vi "Get Board Size.vi"(10 "Board":u32[][](array[colorbox])) -> (1 "Y":i32, 2 "X":i32)   [LabVIEW 2021, in "Board_Game.lvclass"]
uses:
  Board_Game.lvclass
  Board_Game.lvclass/Board_Game.ctl
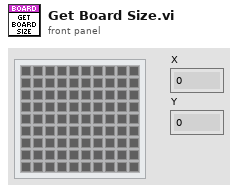
[diagram p1: front panel]
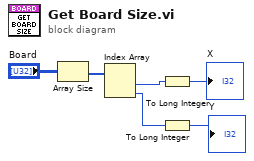
[diagram p0: block diagram]
diagram:
  n1 = Array Size(array="Board") -> (size(s)=w6:i32[])
  n2 = Index Array(array=w6) -> (element #1=w2:i32, element #2=w1:i32)  [unwired: 2 in]
  n3 = To Long Integer(number=w2) -> (32bit integer=→"X":i32)
  n4 = To Long Integer(number=w1) -> (32bit integer=→"Y":i32)
